vi "DELETE Handle setLogData.vi"(8 "error in (no error)":errorcluster, 10 "LogData":variant, 11 "Instrument in":refnum<class "Instrument.lvclass">) -> (0 "error out":errorcluster, 3 "Instrument out":refnum<class "Instrument.lvclass">)   [LabVIEW 2019]
doc: "Override to handle \"getAll\" or \"getAllData\" commands for <b>your</b> Instrument"
uses:
  Instrument.lvclass
  Typedefs/PrivateEvents--Instrument.LogData.ctl
  Instrument.lvclass/Instrument.ctl
  C:/Program Files (x86)/National Instruments/LabVIEW 2019/vi.lib/JKI/JKI SMO/SMO/SMO.lvclass
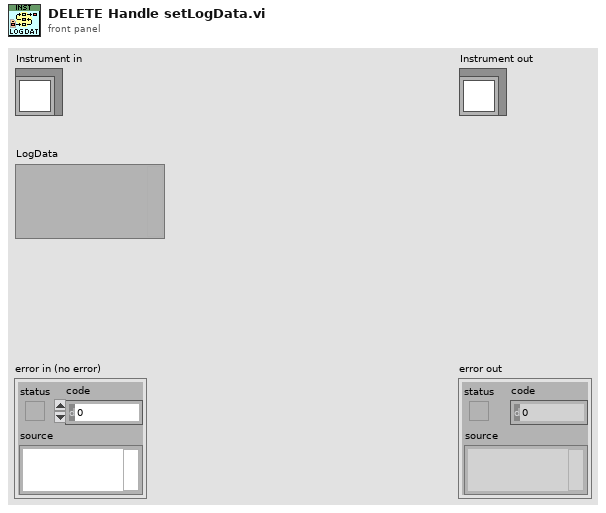
[diagram p1: front panel]
types:
  T1 = typedef "Instrument.lvlib/Instrument.lvclass/PrivateEvents--Instrument.LogData.ctl" = cluster{"path":string, "Data":variant}
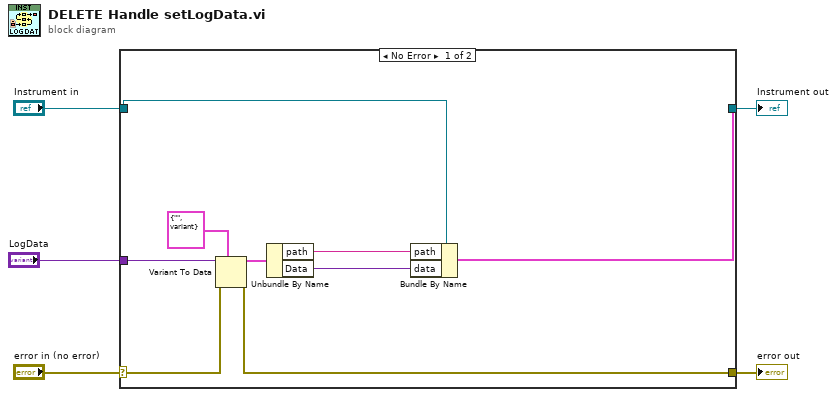
[diagram p0: block diagram]
diagram:
  n1 = case shown="No Error" "error in (no error)" {
    selector: "error in (no error)" -> [w10 w16]
    tunnel: [w9 w16] -> w4
    tunnel: [w14 w15] -> w2
    tunnel: "Instrument in" -> [w13 w15]
    tunnel: "LogData" -> [w11 _]
    frame No Error {
      n2 = Variant To Data(error in=w10, type=T1 {"path"="", "Data"=variant} ("Log Data"), Variant=w11) -> (data=w8:T1, error out=w9:errorcluster)
      n3 = Unbundle By Name(w8) -> ("path"=w7:string, "Data"=w6:variant)
      n4 = Bundle By Name(cluster=w13, "path"=w7, "data"=w6) -> (w14:cluster{})
    }
    frame Error {
    }
  }
  "error out" <- w4
  "Instrument out" <- w2
